vi "CheckEndPack (SubVI).vi"(7 "OptionPACK5":T1={"MagicWordStr"="xV4\u0012", "Header size"=56, "Проверка CRC8"=TRUE, "Проверка конца пакета"=FALSE, "GainCompens"=FALSE, "Неотбрасывать BadEnd пакеты"=TRUE, "Неотбрасывать BadCRC пакеты"=TRUE, "Привести к 1"=FALSE, "GainCoef"=FALSE, "K_scale"=0.0, "ScaleOrdinate"=enum."Проценты"}, 8 "error in":errorcluster, 9 "OfsetEndPack":i32, 11 "data":string="xV4\u0012") -> (0 "error out":errorcluster, 1 "PackToSmall":bool, 2 "PackEndGood":bool)   [LabVIEW 2017]
uses:
  Control_EU/OptionPACK5.ctl
panel:
  out "substring":string
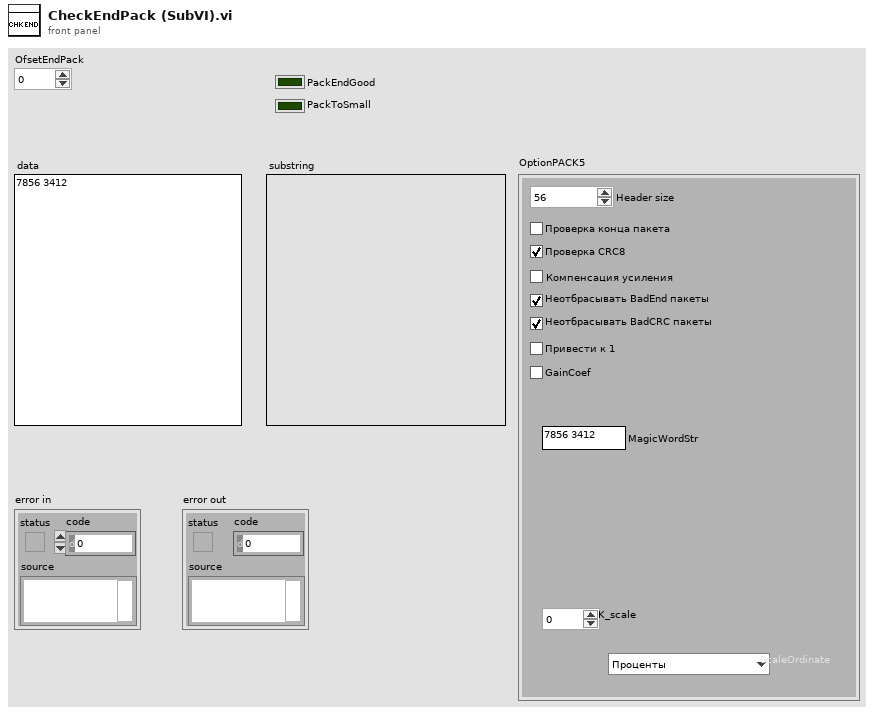
[diagram p1: front panel]
types:
  T1 = typedef "OptionPACK5.ctl" = cluster{"MagicWordStr":string, "Header size":u32, "Проверка CRC8":bool, "Проверка конца пакета":bool, "GainCompens":bool, "Неотбрасывать BadEnd пакеты":bool, "Неотбрасывать BadCRC пакеты":bool, "Привести к 1":bool, "GainCoef":bool, "K_scale":dbl, "ScaleOrdinate":enum16{"Отсчеты АЦП (±32767)", "Проценты", "Вольты", "дБмкВ (отн. 1 мкВ)", "Отсчеты АЦП (±1)"}}
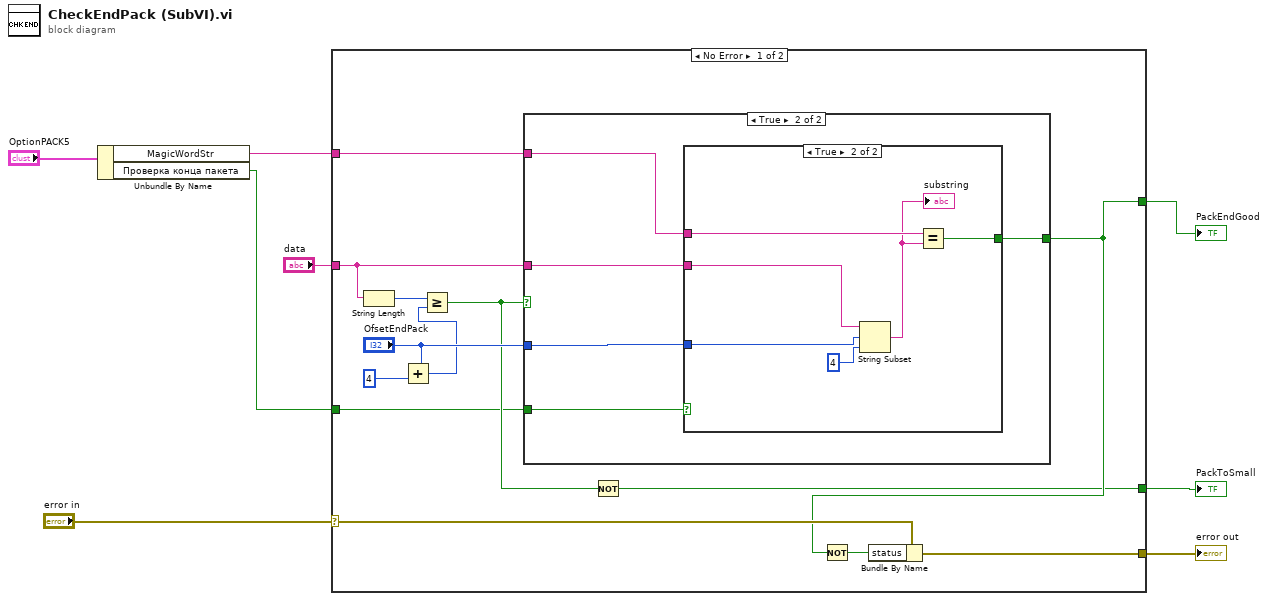
[diagram p0: block diagram]
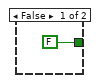
[diagram p2: hidden frame]
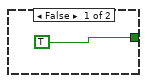
[diagram p3: hidden frame]
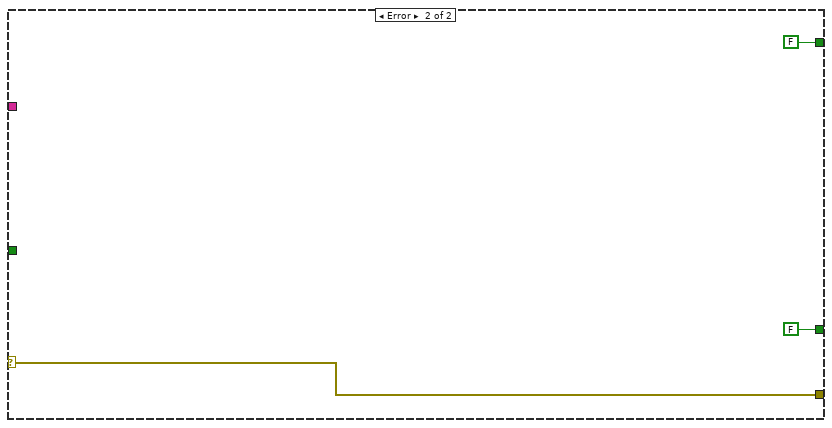
[diagram p4: hidden frame]
diagram:
  n1 = Unbundle By Name("OptionPACK5") -> ("MagicWordStr"=w2:string, "Проверка конца пакета"=w1:bool)
  n2 = case shown="No Error" "error in" {
    selector: "error in" -> [w21 w37]
    tunnel: [w20 w37] -> w7
    tunnel: "data" -> [w17 _]
    tunnel: [w18 FALSE] -> w6
    tunnel: [w12 FALSE] -> w5
    tunnel: w2 -> [w10 _]
    tunnel: w1 -> [w9 _]
    frame No Error {
      n3 = String Length(string=w17) -> (length=w14:i32)
      n4 = Add(x="OfsetEndPack", y=4) -> (x+y=w11:i32)
      n5 = Greater Or Equal?(x=w14, y=w11) -> (x >= y?=w13:bool)
      n6 = case shown="True" w13 {
        tunnel: [FALSE w27] -> w18
        tunnel: w17 -> [_ w26]
        tunnel: "OfsetEndPack" -> [_ w25]
        tunnel: w10 -> [_ w24]
        tunnel: w9 -> [_ w23]
        frame False {
        }
        frame True {
          n7 = case shown="True" w23 {
            tunnel: w25 -> [_ w30]
            tunnel: w26 -> [_ w31]
            tunnel: [TRUE w34] -> w27
            tunnel: w24 -> [_ w33]
            frame False {
            }
            frame True {
              n8 = String Subset(string=w31, offset (0)=w30, length (rest)=4 ("length (rest)")) -> (substring=w32:string)
              "substring" <- w32
              n9 = Equal?(x=w33, y=w32) -> (x = y?=w34:bool)
            }
          }
        }
      }
      n10 = Not(x=w13) -> (.not. x?=w12:bool)
      n11 = Not(x=w18) -> (.not. x?=w19:bool)
      n12 = Bundle By Name(cluster=w21, "status"=w19) -> (w20:errorcluster)
    }
    frame Error {
    }
  }
  "error out" <- w7
  "PackEndGood" <- w6
  "PackToSmall" <- w5
